vi "Magazine_Set.vi"   [LabVIEW 2020]
uses:
  Magazine_Control_States.ctl
  Globals/Magazine_Globals.vi
types:
  T1 = typedef "Magazine_Control_States.ctl" = enum16{"No-Op", "Manual_Control", "Load", "Firing"}
  T2 = typedef "Magazine_Cluster.ctl" = cluster{"Control_States":T1, "Manual_Magazine":dbl, "Load_Magazine":bool, "Firing_Magazine":bool}
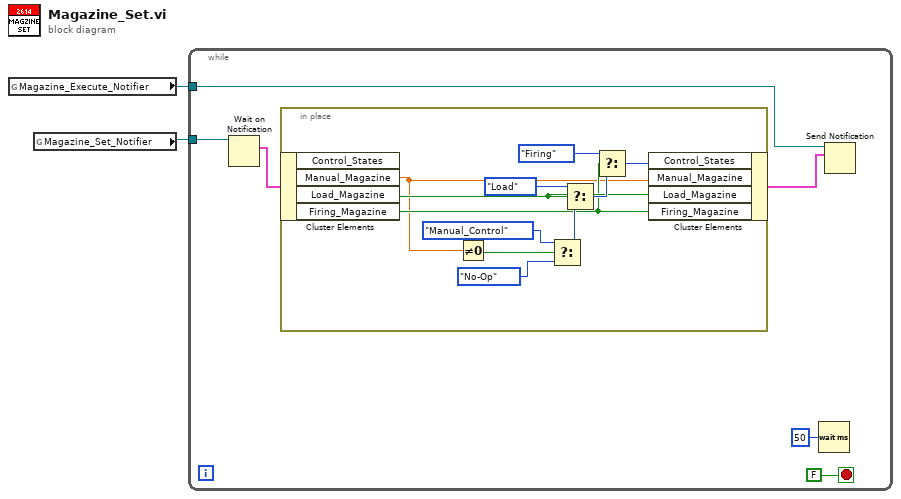
[diagram p0: block diagram]
diagram:
  n1 = global read "Magazine_Globals.vi" "Magazine_Execute_Notifier"() -> (w2:refnum<notifier>)
  n2 = global read "Magazine_Globals.vi" "Magazine_Set_Notifier"() -> (w1:refnum<notifier>)
  n3 = while {
    tunnel: w1 -> [w8]
    tunnel: w2 -> [w4]
    stop <- FALSE stop-if-true
    n4 = Wait on Notification(notifier=w8) -> (notification=w5:T2)  [unwired: 3 in, 3 out]
    n5 = in-place {
      n6 = in-place-cluster #1(w5) -> ("Manual_Magazine"=w9:dbl, "Load_Magazine"=w11:bool, "Firing_Magazine"=w10:bool)  [unwired: 1 out]
      n7 = Not Equal To 0?(x=w9) -> (x != 0?=w17:bool)
      n8 = Select(t=Magazine_Control_States."Manual_Control" ("Control_States"), s=w17, f=Magazine_Control_States."No-Op" ("Control_States")) -> (s? t:f=w16:T1)
      n9 = Select(t=Magazine_Control_States."Load" ("Control_States"), s=w11, f=w16) -> (s? t:f=w14:T1)
      n10 = Select(t=Magazine_Control_States."Firing" ("Control_States"), s=w10, f=w14) -> (s? t:f=w12:T1)
      n11 = in-place-cluster #1("Control_States"=w12, "Manual_Magazine"=w9, "Load_Magazine"=w11, "Firing_Magazine"=w10) -> (w3:T2)
    }
    n12 = Wait (ms)(milliseconds to wait=u32 50) -> ()  [unwired: 1 out]
    n13 = Send Notification(notification=w3, notifier=w4) -> ()  [unwired: 1 in, 2 out]
  }
